vi "MultiChannelFeedbackCooling_aod_feedback(Host)_PIDXYZ_laserPID.vi"(5 "RIO Device":T1="RIO0") -> ()   [LabVIEW 2018]
doc: "This VI will will initialize the FPGA VI and then continually read and convert single point values from 4 channels of an analog input module."
uses:
  <vilib>/userdefined/High Color/nirio_resource_hc.ctl
  <vilib>/rvi/Analysis/host/Butterworth/config/Butterworth Filter Order.ctl
  <vilib>/rvi/Analysis/host/Butterworth/config/Butterworth Filter Type.ctl
  <vilib>/FPGAPlugInAG/PXIe-7856R/niLvFpga_Open_PXIe-7856R.vi
  <vilib>/FPGAPlugInAG/PXIe-7856R/niLvFpga_Run_PXIe-7856R.vi
  <vilib>/rvi/Analysis/host/Butterworth/config/BwScaledCoefficients.vi
  <vilib>/Utility/error.llb/Error Cluster From Error Code.vi
  <vilib>/rvi/errors/niLvFpgaAdjustHostInterfaceError.vi
  <vilib>/Utility/file.llb/Read From Spreadsheet File (I64).vi
  <vilib>/FPGAPlugInAG/PXIe-7856R/niLvFpga_Close_PXIe-7856R.vi
  <vilib>/rvi/interface/nirviOpenFPGA/nirviOpenFPGA.xnode
  FPGA Bitfiles/Microspherefeedb_FPGATarget2_MultiChannelfFee_SMENcAWM-fA.lvbitx
  <vilib>/rvi/interface/nirviMethod/nirviMethod.xnode
  <vilib>/rvi/Analysis/host/Butterworth/XNode/ButterworthCoefficients.xnode
  <vilib>/rvi/interface/nirviReadWriteControl/nirviReadWriteControl.xnode
  <vilib>/rvi/interface/nirviCloseFPGA/nirviCloseFPGA.xnode
  NiFpgaLv.dll
  <vilib>/rvi/Analysis/host/Public/NI_FpgaMspHost.lvlib
panel:
  in  "LP FF Z before":dbl=1000.0
  in  "LP FF Y before":dbl=1000.0
  in  "LP FF X Before":dbl=1000.0
  in  "LP FF Z":dbl=5000.0
  in  "LP FF Y":dbl=5000.0
  in  "LP FF X":dbl=5000.0
  in  "Lower lim Y before":fxp<+/-,16,16>=10000.0
  in  "Upper lim Y before":fxp<+/-,16,16>=10000.0
  in  "Lower lim X before":fxp<+/-,16,16>=10000.0
  in  "Upper lim X before":fxp<+/-,16,16>=10000.0
  in  "?":u16(ring)=2 items=["Both", "AOD", "Bead"]
  in  "?":u16(ring)=2 items=["Both", "AOD", "Bead"]
  out "Tot feedback + DC, Z":i16(graph)=16788
  out "Individual feedback, Z":cluster{"fb_0":i16, "fb_d0":i16}(graph)
  out "AI 2":cluster{"AI1":i16, "AI4":i16}(graph)={"AI1"=5242, "AI4"=5242}
  in  "Use PID Y before":bool
  in  "Use PID X before":bool
  in  "Ig Y before":fxp<+/-,24,12>
  in  "Dg Y before":fxp<+/-,24,12>
  in  "Pg Y before":fxp<+/-,24,12>
  in  "Ig X before":fxp<+/-,24,12>
  in  "Dg X before":fxp<+/-,24,12>
  in  "Pg X before":fxp<+/-,24,12>
  in  "Y before setpoint":i16
  in  "X before setpoint":i16
  in  "dg band X before":fxp<+/-,24,12>
  in  "dg band Y before":fxp<+/-,24,12>
  in  "hp freq X band before":dbl=5000.0
  in  "lp freq X band before":dbl=5000.0
  in  "hp freq X before":dbl=5000.0
  in  "lp freq X before":dbl=5000.0
  in  "hp freq Y band before":dbl=5000.0
  in  "lp freq Y band before":dbl=5000.0
  in  "hp freq Y before":dbl=5000.0
  in  "lp freq Y before":dbl=5000.0
  out "EOM_amplitude_out":dbl=4.999694842844065
  in  "EOM_offset (-10 to 10 V)":dbl
  in  "EOM_amplitude (-10 to 10 V)":dbl=5.0
  in  "EOM_threshold (0 to 1), (2*thr - 1)*ampli":dbl=1.0
  in  "EOM reset":bool
  in  "hp freq band Z before":dbl=5000.0
  in  "lp freq band Z before":dbl=5000.0
  in  "dg band Z before":fxp<+/-,24,12>
  in  "hp freq bandZ":dbl=49.0
  in  "lp freq bandZ":dbl=45.0
  in  "dg band Z":fxp<+/-,24,12>
  in  "dg band Y":fxp<+/-,24,12>
  in  "hp freq bandY":dbl=5000.0
  in  "lp freq bandY":dbl=5000.0
  in  "hp freq bandX":dbl=5000.0
  in  "lp freq bandX":dbl=5000.0
  in  "dg band X":fxp<+/-,24,12>
  in  "Pg Y":fxp<+/-,24,12>
  in  "Ig Y":fxp<+/-,24,6>
  in  "Pg X":fxp<+/-,24,12>
  in  "Ig X":fxp<+/-,24,6>
  in  "End value arb (ch1)":fxp<+/-,32,16>=1.0
  in  "Step arb (ch1)":fxp<+/-,32,16>=0.100006103515625
  in  "Arb gain (Z)":fxp<+/-,24,12>=1.0
  in  "z arb scale":fxp<+/-,33,17>=1.0
  in  "ramp arb drive":bool
  in  "End value arb (ch0)":fxp<+/-,32,16>=1.0
  in  "Step arb (ch0)":fxp<+/-,32,16>=1.0
  in  "Delay Time (s) arb":dbl=0.001 caption="Delay Time (s)"
  in  "Buffer file path":path=path "C:/Users/yalem/GitHub/Documents/Optlev/scriptssiny_buffer.txt"
  in  "Write data to buffers":bool
  in  "Arb steps per cycle":u16=20
  in  "Arb gain (Y)":fxp<+/-,24,12>
  in  "Arb gain (X)":fxp<+/-,24,12>
  in  "Z before setpoint":i16
  in  "Upper lim Z before":fxp<+/-,16,16>=10000.0
  in  "Lower lim Z before":fxp<+/-,16,16>=-10000.0
  in  "hp freq Z before":dbl=5000.0
  in  "lp freq Z before":dbl=5000.0
  in  "Use PID Z before":bool
  in  "hp freq Y":dbl=1300.0
  in  "hp freq X":dbl=1300.0
  in  "lp freq X":dbl=1300.0
  in  "DC offset X":i16=16310
  in  "Lower lim X":fxp<+/-,16,16>=-15000.0
  in  "Upper lim X":fxp<+/-,16,16>=15000.0
  in  "Dg X":fxp<+/-,24,12>
  in  "X setpoint":i16
  in  "change pars":bool
  in  "hp freq Z":dbl=1800.0
  in  "lp freq Y":dbl=1300.0
  in  "lp freq Z":dbl=1800.0
  in  "ramp power":bool
  in  "End value power":i16=10200
  in  "Step power":i16=4
  in  "Delay Time (s) power":dbl=0.01 caption="Delay Time (s)"
  in  "Count(usec)":u32=10
  in  "?":u16(ring)=2 items=["Both", "AOD", "Bead"]
  in  "?":u16(ring)=2 items=["Both", "AOD", "Bead"]
  in  "?":u16(ring)=2 items=["Both", "AOD", "Bead"]
  in  "?":u16(ring)=2 items=["Both", "AOD", "Bead"]
  in  "Pg Z before":fxp<+/-,24,12>
  in  "Ig Z before":fxp<+/-,24,6>
  in  "Dg Z before":fxp<+/-,24,12>
  in  "Ig Z":fxp<+/-,24,6>
  in  "DC offset Z":i16=16788
  in  "Lower lim Z":fxp<+/-,16,16>=-20.0
  in  "Upper lim Z":fxp<+/-,16,16>=1000.0
  in  "Dg Z":fxp<+/-,24,12>
  in  "Pg Z":fxp<+/-,24,12>
  in  "Z setpoint":i16
  in  "change pars 2":bool
  in  "change pars 1":bool
  in  "DC offset Y":i16=16310
  in  "Lower lim Y":fxp<+/-,16,16>=-15000.0
  in  "Upper lim Y":fxp<+/-,16,16>=15000.0
  in  "Dg Y":fxp<+/-,24,12>
  in  "Y setpoint":i16
  out "Tot feedback + DC, Y":i16(graph)=16310
  out "Individual feedback, Y":cluster{"fb_0":i16, "fb_d0":i16}(graph)
  out "AI1":cluster{"AI1":i16, "AI4":i16}(graph)={"AI1"=-2712, "AI4"=-2712}
  out "Tot feedback + DC, X":i16(graph)=16309
  out "Individual feedback, X":cluster{"fb_0":i16, "fb_d0":i16}(graph)
  out "AI0":cluster{"AI0":i16, "AI3":i16}(graph)={"AI0"=-863, "AI3"=-863}
  in  "stop":bool
  # "FPGA feedback GUI"
  # "Bead arbitrary drive:"
  # "PID controls, X (ch 0):"
  # "Bead feedback:"
  # "PID controls, Y (ch 1):"
  # "Bead feedback:"
  # "PID controls, Z (ch 2):"
  # "Bead feedback:"
  # "AOD feeback:"
types:
  T1 = typedef "nirio_resource_hc.ctl" = tag
  T2 = cluster{"fb Z plot":i16, "fb Z before chamber plot":i16}
  T3 = cluster{"fb Z before chamber plot":i16, "fb Z before chamber plot":i16}
  T4 = cluster{"AI Z plot":i16, "AI Z before chamber plot":i16}
  T5 = cluster{"AI Z before chamber plot":i16, "AI Z before chamber plot":i16}
  T6 = cluster{"AI X plot":i16, "AI X before chamber plot":i16}
  T7 = cluster{"AI X before chamber plot":i16, "AI X before chamber plot":i16}
  T8 = cluster{"fb X plot":i16, "fb X before chamber plot":i16}
  T9 = cluster{"fb X before chamber plot":i16, "fb X before chamber plot":i16}
  T10 = cluster{"fb Y plot":i16, "fb Y before chamber plot":i16}
  T11 = cluster{"fb Y before chamber plot":i16, "fb Y before chamber plot":i16}
  T12 = cluster{"AI Y plot":i16, "AI Y before chamber plot":i16}
  T13 = cluster{"AI Y before chamber plot":i16, "AI Y before chamber plot":i16}
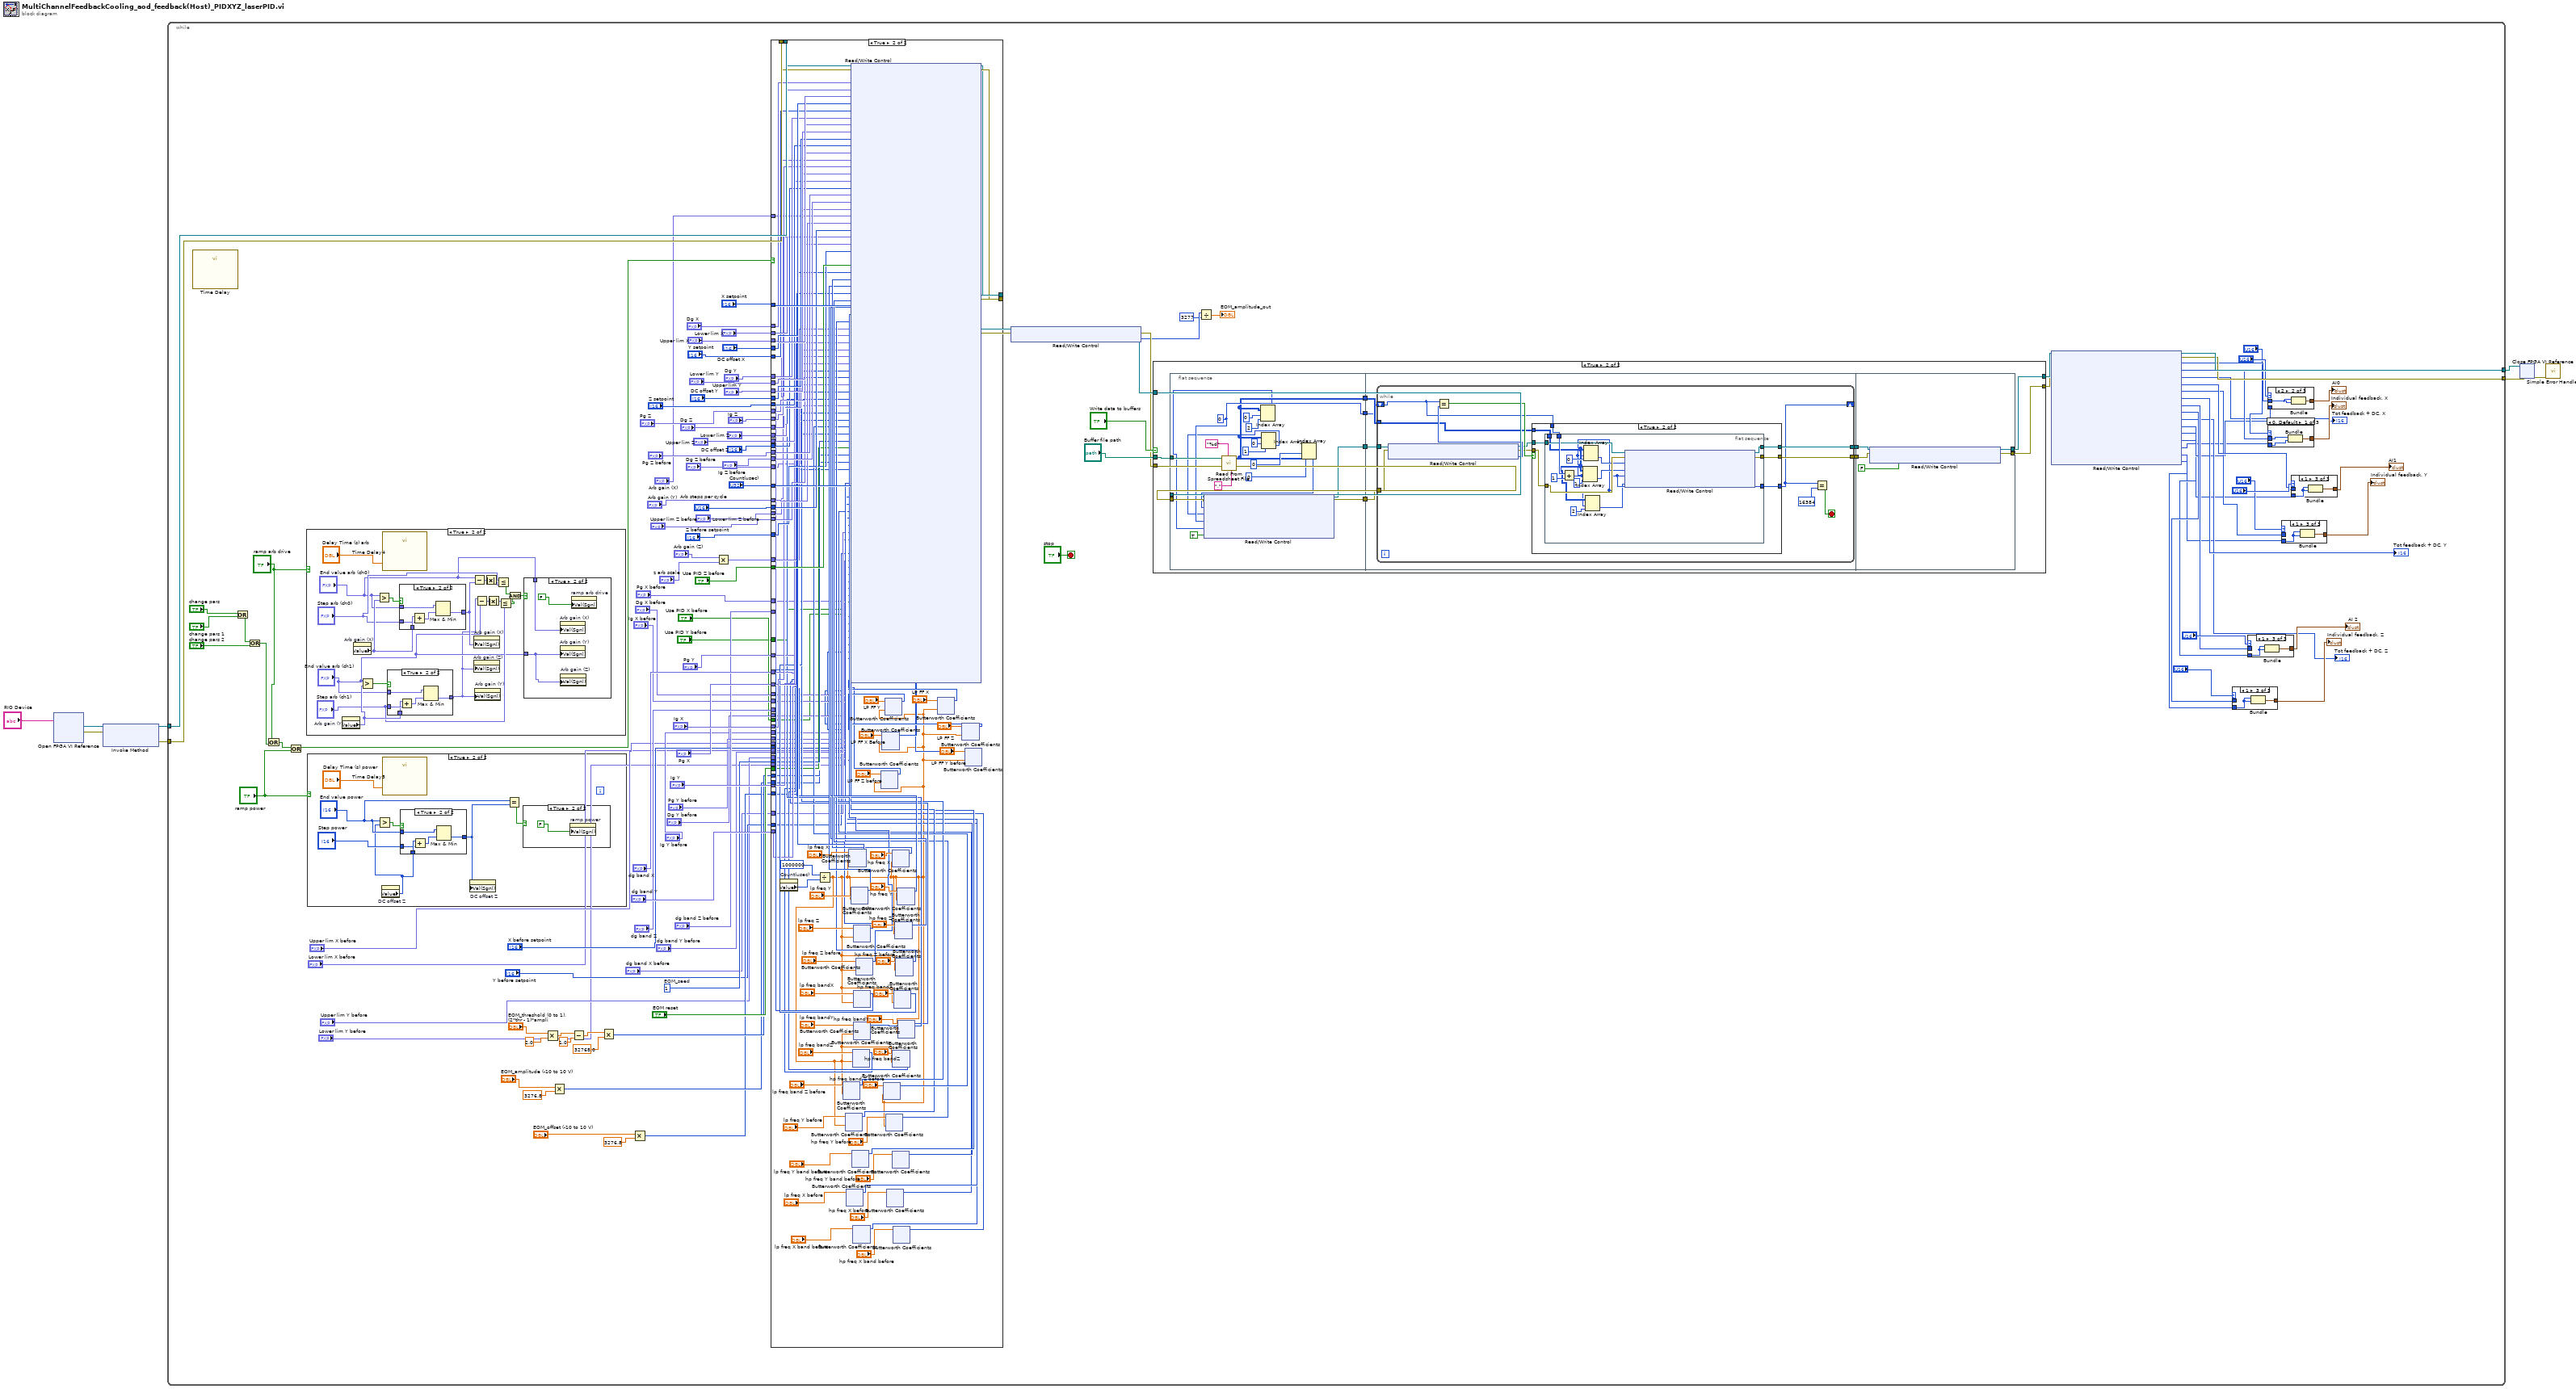
[diagram p0: block diagram]
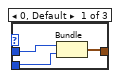
[diagram p2: hidden frame]
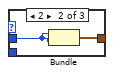
[diagram p3: hidden frame]
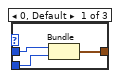
[diagram p4: hidden frame]
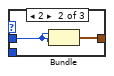
[diagram p5: hidden frame]
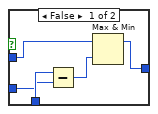
[diagram p8: hidden frame]
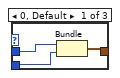
[diagram p9: hidden frame]
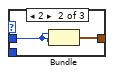
[diagram p10: hidden frame]
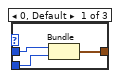
[diagram p11: hidden frame]
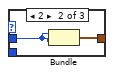
[diagram p12: hidden frame]
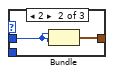
[diagram p13: hidden frame]
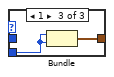
[diagram p14: hidden frame]
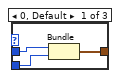
[diagram p15: hidden frame]
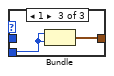
[diagram p16: hidden frame]
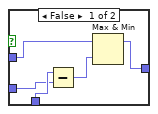
[diagram p18: hidden frame]
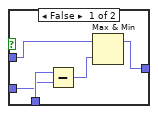
[diagram p20: hidden frame]
diagram:
  n1 = xnode "Open FPGA VI Reference"("resource name"="RIO Device") -> ("FPGA VI Reference Out"=w3:refnum<k20>, "error out"=w2:errorcluster)  [unwired: 1 in]
  n2 = xnode "Invoke Method"("FPGA VI Reference In"=w3, "error in"=w2) -> ("FPGA VI Reference Out"=w5:refnum<k20>, "error out"=w4:errorcluster)  [unwired: 1 in]
  n3 = while {
    tunnel: [w130] -> w8
    tunnel: w5 -> [w122]
    tunnel: w4 -> [w121]
    tunnel: [w129] -> w1
    stop <- "stop" stop-if-true
    w60 = u32 1  # EOM_seed
    n4 = call "Time Delay"() -> ()  [unwired: 11 in, 1 out]
    n5 = Or(x="change pars", y="change pars 1") -> (x .or. y?=w97:bool)
    n6 = Or(x=w97, y="change pars 2") -> (x .or. y?=w73:bool)
    n7 = Or(x="ramp arb drive", y=w73) -> (x .or. y?=w80:bool)
    n8 = Or(x=w80, y="ramp power") -> (x .or. y?=w81:bool)
    n9 = case shown="True" "ramp arb drive" {
      frame False {
      }
      frame True {
        n10 = property on="Arb gain (Y)" class="DigNum (strict)"() -> ("Value"=w204:fxp<+/-,24,12>)  [unwired: 2 in, 2 out]
        n11 = property on="Arb gain (X)" class="DigNum (strict)"() -> ("Value"=w207:fxp<+/-,24,12>)  [unwired: 2 in, 2 out]
        n12 = Greater?(x="End value arb (ch1)", y=w204) -> (0:w205:bool)
        n13 = Greater?(x="End value arb (ch0)", y=w207) -> (0:w208:bool)
        n14 = call "Time Delay4"("Delay Time (s)"="Delay Time (s) arb") -> ()  [unwired: 10 in, 1 out]
        n15 = case shown="True" w205 {
          tunnel: "End value arb (ch1)" -> [w210 w216]
          tunnel: w204 -> [w213 w214]
          tunnel: "Step arb (ch1)" -> [w212 w218]
          tunnel: [w209 w215] -> w191
          frame False {
            n16 = Subtract(x=w213, y=w212) -> (x-y=w211:fxp<+/-,33,17>)
            n17 = Max & Min(x=w210, y=w211) -> (max(x,y)=w209:fxp<+/-,33,17>)  [unwired: 1 out]
          }
          frame True {
            n18 = Add(x=w214, y=w218) -> (x+y=w217:fxp<+/-,33,17>)
            n19 = Max & Min(x=w216, y=w217) -> (min(x,y)=w215:fxp<+/-,33,17>)  [unwired: 1 out]
          }
        }
        n20 = case shown="True" w208 {
          tunnel: "End value arb (ch0)" -> [w223 w228]
          tunnel: w207 -> [w226 w231]
          tunnel: "Step arb (ch0)" -> [w225 w230]
          tunnel: [w222 w227] -> w203
          frame False {
            n21 = Subtract(x=w226, y=w225) -> (x-y=w224:fxp<+/-,33,17>)
            n22 = Max & Min(x=w223, y=w224) -> (max(x,y)=w222:fxp<+/-,33,17>)  [unwired: 1 out]
          }
          frame True {
            n23 = Add(x=w231, y=w230) -> (x+y=w229:fxp<+/-,33,17>)
            n24 = Max & Min(x=w228, y=w229) -> (min(x,y)=w227:fxp<+/-,33,17>)  [unwired: 1 out]
          }
        }
        n25 = Subtract(x="End value arb (ch0)", y=w203) -> (x-y=w202:fxp<+/-,34,18>)
        n26 = property on="Arb gain (X)" class="DigNum (strict)"("Val(Sgnl)"=w203) -> ()  [unwired: 2 in, 2 out]
        n27 = property on="Arb gain (Z)" class="DigNum (strict)"("Val(Sgnl)"=w191) -> ()  [unwired: 2 in, 2 out]
        n28 = Subtract(x=w191, y="End value arb (ch1)") -> (x-y=w199:fxp<+/-,34,18>)
        n29 = property on="Arb gain (Y)" class="DigNum (strict)"("Val(Sgnl)"=w191) -> ()  [unwired: 2 in, 2 out]
        n30 = Absolute Value(x=w202) -> (abs(x)=w201:fxp<+,33,17>)
        n31 = Absolute Value(x=w199) -> (abs(x)=w198:fxp<+,33,17>)
        n32 = Less Or Equal?(x=w201, y="Step arb (ch0)") -> (x <= y?=w195:bool)
        n33 = Less Or Equal?(x=w198, y="Step arb (ch1)") -> (x <= y?=w194:bool)
        n34 = And(x=w195, y=w194) -> (x .and. y?=w196:bool)
        n35 = case shown="True" w196 {
          tunnel: "End value arb (ch0)" -> [_ w220]
          tunnel: "End value arb (ch1)" -> [_ w219]
          frame False {
          }
          frame True {
            n36 = property on="Arb gain (X)" class="DigNum (strict)"("Val(Sgnl)"=w220) -> ()  [unwired: 2 in, 2 out]
            n37 = property on="Arb gain (Y)" class="DigNum (strict)"("Val(Sgnl)"=w219) -> ()  [unwired: 2 in, 2 out]
            n38 = property on="Arb gain (Z)" class="DigNum (strict)"("Val(Sgnl)"=w219) -> ()  [unwired: 2 in, 2 out]
            n39 = property on="ramp arb drive" class="Bool (strict)"("Val(Sgnl)"=FALSE) -> ()  [unwired: 2 in, 2 out]
          }
        }
      }
    }
    n40 = case shown="True" "ramp power" {
      frame False {
      }
      frame True {
        n41 = property on="DC offset Z" class="DigNum (strict)"() -> ("Value"=w146:i16)  [unwired: 2 in, 2 out]
        n42 = Greater?(x="End value power", y=w146) -> (0:w151:bool)
        n43 = call "Time Delay5"("Delay Time (s)"="Delay Time (s) power") -> ()  [unwired: 10 in, 1 out]
        n44 = case shown="True" w151 {
          tunnel: "End value power" -> [w154 w159]
          tunnel: w146 -> [w157 w162]
          tunnel: "Step power" -> [w156 w161]
          tunnel: [w153 w158] -> w145
          frame False {
            n45 = Subtract(x=w157, y=w156) -> (x-y=w155:i16)
            n46 = Max & Min(x=w154, y=w155) -> (max(x,y)=w153:i16)  [unwired: 1 out]
          }
          frame True {
            n47 = Add(x=w162, y=w161) -> (x+y=w160:i16)
            n48 = Max & Min(x=w159, y=w160) -> (min(x,y)=w158:i16)  [unwired: 1 out]
          }
        }
        n49 = property on="DC offset Z" class="DigNum (strict)"("Val(Sgnl)"=w145) -> ()  [unwired: 2 in, 2 out]
        n50 = Equal?(x="End value power", y=w145) -> (x = y?=w150:bool)
        n51 = case shown="True" w150 {
          frame False {
          }
          frame True {
            n52 = property on="ramp power" class="Bool (strict)"("Val(Sgnl)"=FALSE) -> ()  [unwired: 2 in, 2 out]
          }
        }
      }
    }
    n53 = Multiply(x="EOM_threshold (0 to 1), (2*thr - 1)*ampli", y=2.0) -> (x*y=w56:dbl)
    n54 = Multiply(x="EOM_amplitude (-10 to 10 V)", y=3276.8) -> (x*y=w49:i16)
    n55 = Subtract(x=w56, y=1.0) -> (x-y=w54:dbl)
    n56 = Multiply(x=w54, y=32768.0) -> (x*y=w52:i16)
    n57 = Multiply(x="EOM_offset (-10 to 10 V)", y=3276.8) -> (x*y=w46:i16)
    n58 = Multiply(x="Arb gain (Z)", y="z arb scale") -> (x*y=w70:fxp<+/-,56,28>)
    n59 = case shown="True" w81 {
      tunnel: w121 -> [w313 w429]
      tunnel: [w313 w437] -> w45
      tunnel: [w312 w436] -> w44
      tunnel: "X setpoint" -> [_ w435]
      tunnel: "Dg X" -> [_ w434]
      tunnel: "Upper lim X" -> [_ w432]
      tunnel: "Lower lim X" -> [_ w433]
      tunnel: "DC offset X" -> [_ w431]
      tunnel: w122 -> [w312 w430]
      tunnel: "Y setpoint" -> [_ w428]
      tunnel: "Dg Y" -> [_ w427]
      tunnel: "Lower lim Y" -> [_ w426]
      tunnel: "Upper lim Y" -> [_ w425]
      tunnel: "DC offset Y" -> [_ w424]
      tunnel: "Z setpoint" -> [_ w423]
      tunnel: "Pg Z" -> [_ w422]
      tunnel: "Ig Z" -> [_ w421]
      tunnel: "Dg Z" -> [_ w420]
      tunnel: "Lower lim Z" -> [_ w419]
      tunnel: "Upper lim Z" -> [_ w418]
      tunnel: "DC offset Z" -> [_ w417]
      tunnel: "Pg Z before" -> [_ w416]
      tunnel: "Ig Z before" -> [_ w415]
      tunnel: "Dg Z before" -> [_ w360]
      tunnel: "Arb gain (Y)" -> [_ w401]
      tunnel: "Arb steps per cycle" -> [_ w414]
      tunnel: "Count(usec)" -> [_ w413]
      tunnel: "Use PID Z before" -> [_ w404]
      tunnel: "Lower lim Z before" -> [_ w400]
      tunnel: "Upper lim Z before" -> [_ w399]
      tunnel: "Z before setpoint" -> [_ w398]
      tunnel: w70 -> [_ w389]
      tunnel: "Ig X" -> [_ w388]
      tunnel: "Pg X" -> [_ w387]
      tunnel: "Ig Y" -> [_ w386]
      tunnel: "Pg Y" -> [_ w385]
      tunnel: "dg band X" -> [_ w384]
      tunnel: "dg band Y" -> [_ w377]
      tunnel: "dg band Z" -> [_ w374]
      tunnel: "dg band Z before" -> [_ _]
      tunnel: w60 -> [_ w365]
      tunnel: "EOM reset" -> [_ w364]
      tunnel: w52 -> [_ w363]
      tunnel: w49 -> [_ w362]
      tunnel: w46 -> [_ w361]
      tunnel: "dg band Y before" -> [_ w343]
      tunnel: "dg band X before" -> [_ w342]
      tunnel: "X before setpoint" -> [_ w341]
      tunnel: "Y before setpoint" -> [_ w340]
      tunnel: "Pg X before" -> [_ w339]
      tunnel: "Dg X before" -> [_ w338]
      tunnel: "Ig X before" -> [_ w337]
      tunnel: "Pg Y before" -> [_ w336]
      tunnel: "Dg Y before" -> [_ w335]
      tunnel: "Ig Y before" -> [_ w334]
      tunnel: "Use PID X before" -> [_ w333]
      tunnel: "Use PID Y before" -> [_ w332]
      tunnel: "Upper lim X before" -> [_ w331]
      tunnel: "Lower lim X before" -> [_ w330]
      tunnel: "Upper lim Y before" -> [_ w329]
      tunnel: "Lower lim Y before" -> [_ w328]
      tunnel: "Arb gain (X)" -> [_ w314]
      frame False {
      }
      frame True {
        n60 = property on="Count(usec)" class="DigNum (strict)"() -> ("Value"=w409:u32)  [unwired: 2 in, 2 out]
        n61 = Divide(x=u32 1000000, y=w409) -> (x/y=w316:dbl)
        n62 = xnode "Butterworth Coefficients"("cutoff frequency (Hz)"="lp freq band Z before", "sample rate (S/s)"=w316) -> ("scaled coefficients"=w366:i32[])  [unwired: 1 in, 1 out]
        n63 = xnode "Butterworth Coefficients"("cutoff frequency (Hz)"="lp freq Y before", "sample rate (S/s)"=w316) -> ("scaled coefficients"=w357:i32[])  [unwired: 1 in, 1 out]
        n64 = xnode "Butterworth Coefficients"("cutoff frequency (Hz)"="lp freq X before") -> ("scaled coefficients"=w347:i32[])  [unwired: 2 in, 1 out]
        n65 = xnode "Butterworth Coefficients"("cutoff frequency (Hz)"="lp freq X", "sample rate (S/s)"=w316) -> ("scaled coefficients"=w397:i32[])  [unwired: 1 in, 1 out]
        n66 = xnode "Butterworth Coefficients"("cutoff frequency (Hz)"="lp freq Y", "sample rate (S/s)"=w316) -> ("scaled coefficients"=w395:i32[])  [unwired: 1 in, 1 out]
        n67 = xnode "Butterworth Coefficients"("cutoff frequency (Hz)"="lp freq Y band before") -> ("scaled coefficients"=w353:i32[])  [unwired: 2 in, 1 out]
        n68 = xnode "Butterworth Coefficients"("cutoff frequency (Hz)"="lp freq bandZ", "sample rate (S/s)"=w316) -> ("scaled coefficients"=w370:i32[])  [unwired: 1 in, 1 out]
        n69 = xnode "Butterworth Coefficients"("cutoff frequency (Hz)"="lp freq X band before") -> ("scaled coefficients"=w345:i32[])  [unwired: 2 in, 1 out]
        n70 = xnode "Butterworth Coefficients"("cutoff frequency (Hz)"="lp freq Z", "sample rate (S/s)"=w316) -> ("scaled coefficients"=w393:i32[])  [unwired: 1 in, 1 out]
        n71 = xnode "Butterworth Coefficients"("cutoff frequency (Hz)"="lp freq bandX", "sample rate (S/s)"=w316) -> ("scaled coefficients"=w380:i32[])  [unwired: 1 in, 1 out]
        n72 = xnode "Butterworth Coefficients"("cutoff frequency (Hz)"="lp freq bandY", "sample rate (S/s)"=w316) -> ("scaled coefficients"=w376:i32[])  [unwired: 1 in, 1 out]
        n73 = xnode "Butterworth Coefficients"("cutoff frequency (Hz)"="lp freq Z before", "sample rate (S/s)"=w316) -> ("scaled coefficients"=w391:i32[])  [unwired: 1 in, 1 out]
        n74 = xnode "Butterworth Coefficients"("cutoff frequency (Hz)"="LP FF Z before", "sample rate (S/s)"=w316) -> ("scaled coefficients"=w315:i32[])  [unwired: 1 in, 1 out]
        n75 = xnode "Butterworth Coefficients"("cutoff frequency (Hz)"="LP FF X Before", "sample rate (S/s)"=w316) -> ("scaled coefficients"=w320:i32[])  [unwired: 1 in, 1 out]
        n76 = xnode "Butterworth Coefficients"("cutoff frequency (Hz)"="hp freq band Z before", "sample rate (S/s)"=w316) -> ("scaled coefficients"=w367:i32[])  [unwired: 1 in, 1 out]
        n77 = xnode "Butterworth Coefficients"("cutoff frequency (Hz)"="LP FF Y", "sample rate (S/s)"=w316) -> ("scaled coefficients"=w324:i32[])  [unwired: 1 in, 1 out]
        n78 = xnode "Butterworth Coefficients"("cutoff frequency (Hz)"="hp freq Y before", "sample rate (S/s)"=w316) -> ("scaled coefficients"=w356:i32[])  [unwired: 1 in, 1 out]
        n79 = xnode "Butterworth Coefficients"("cutoff frequency (Hz)"="hp freq X before") -> ("scaled coefficients"=w346:i32[])  [unwired: 2 in, 1 out]
        n80 = xnode "Butterworth Coefficients"("cutoff frequency (Hz)"="hp freq X", "sample rate (S/s)"=w316) -> ("scaled coefficients"=w396:i32[])  [unwired: 1 in, 1 out]
        n81 = xnode "Butterworth Coefficients"("cutoff frequency (Hz)"="hp freq Y band before") -> ("scaled coefficients"=w352:i32[])  [unwired: 2 in, 1 out]
        n82 = xnode "Butterworth Coefficients"("cutoff frequency (Hz)"="hp freq bandZ", "sample rate (S/s)"=w316) -> ("scaled coefficients"=w371:i32[])  [unwired: 1 in, 1 out]
        n83 = xnode "Butterworth Coefficients"("cutoff frequency (Hz)"="hp freq X band before") -> ("scaled coefficients"=w344:i32[])  [unwired: 2 in, 1 out]
        n84 = xnode "Butterworth Coefficients"("cutoff frequency (Hz)"="hp freq bandX", "sample rate (S/s)"=w316) -> ("scaled coefficients"=w381:i32[])  [unwired: 1 in, 1 out]
        n85 = xnode "Butterworth Coefficients"("cutoff frequency (Hz)"="hp freq Z", "sample rate (S/s)"=w316) -> ("scaled coefficients"=w392:i32[])  [unwired: 1 in, 1 out]
        n86 = xnode "Butterworth Coefficients"("cutoff frequency (Hz)"="hp freq Z before", "sample rate (S/s)"=w316) -> ("scaled coefficients"=w390:i32[])  [unwired: 1 in, 1 out]
        n87 = xnode "Butterworth Coefficients"("cutoff frequency (Hz)"="hp freq Y", "sample rate (S/s)"=w316) -> ("scaled coefficients"=w394:i32[])  [unwired: 1 in, 1 out]
        n88 = xnode "Butterworth Coefficients"("cutoff frequency (Hz)"="hp freq bandY", "sample rate (S/s)"=w316) -> ("scaled coefficients"=w375:i32[])  [unwired: 1 in, 1 out]
        n89 = xnode "Butterworth Coefficients"("cutoff frequency (Hz)"="LP FF X", "sample rate (S/s)"=w316) -> ("scaled coefficients"=w326:i32[])  [unwired: 1 in, 1 out]
        n90 = xnode "Butterworth Coefficients"("cutoff frequency (Hz)"="LP FF Z", "sample rate (S/s)"=w316) -> ("scaled coefficients"=w322:i32[])  [unwired: 1 in, 1 out]
        n91 = xnode "Butterworth Coefficients"("cutoff frequency (Hz)"="LP FF Y before", "sample rate (S/s)"=w316) -> ("scaled coefficients"=w318:i32[])  [unwired: 1 in, 1 out]
        n92 = xnode "Read/Write Control"("FPGA VI Reference In"=w430, "error in"=w429, "X Setpoint"=w435, "dg X"=w434, "Lower lim X"=w433, "Upper lim X"=w432, "DC offset X"=w431, "Y Setpoint"=w428, "dg Y"=w427, "Lower lim Y"=w426, "Upper lim Y"=w425, "DC offset Y"=w424, "Z Setpoint"=w423, "pg Z"=w422, "ig Z"=w421, "dg Z"=w420, "Lower lim Z"=w419, "Upper lim Z"=w418, "DC offset Z"=w417, "pg Z before"=w416, "ig Z before"=w415, "dg Z before"=w360, "Arb gain (ch0)"=w314, "Arb gain (ch1)"=w401, "Arb steps per cycle"=w414, "Lower lim Z before"=w400, "Upper lim Z before"=w399, "Z before Setpoint"=w398, "Count(uSec)"=w413, "Use Z PID before"=w404, "LP Coeff X"=w397, "HP Coeff X"=w396, "LP Coeff Y"=w395, "HP Coeff Y"=w394, "LP Coeff Z"=w393, "HP Coeff Z"=w392, "LP Coeff band Z before"=w391, "HP coeff band Z before"=w390, "Arb gain (ch2)"=w389, "ig X"=w388, "pg X"=w387, "ig Y"=w386, "pg Y"=w385, "dg band X"=w384, "HP Coeff band X"=w381, "LP Coeff band X"=w380, "dg band Y"=w377, "HP Coeff band Y"=w375, "LP Coeff band Y"=w376, "dg band Z"=w374, "HP Coeff band Z"=w371, "LP Coeff band Z"=w370, "HP Coeff band Z"=w367, "LP Coeff band Z"=w366, "EOM_seed"=w365, "EOM reset"=w364, "EOM_threshold"=w363, "EOM_amplitude"=w362, "EOM_offset"=w361, "LP Coeff Y before"=w357, "HP Coeff Y before"=w356, "LP Coeff band Y before"=w353, "HP coeff band Y before"=w352, "LP Coeff X before"=w347, "HP Coeff X before"=w346, "LP Coeff band X before"=w345, "HP coeff band X before"=w344, "dg band Y before"=w343, "dg band X before"=w342, "X before Setpoint"=w341, "Y before Setpoint"=w340, "pg X before"=w339, "dg X before"=w338, "ig X before"=w337, "pg Y before"=w336, "dg Y before"=w335, "ig Y before"=w334, "Use X PID before"=w333, "Use Y PID before"=w332, "Upper lim X before"=w331, "Lower lim X before"=w330, "Upper lim Y before"=w329, "Lower lim Y before"=w328, "final filter coeff X"=w326, "final filter coeff Y"=w324, "final filter coeff Z"=w322, "final filter coeff X before"=w320, "final filter coeff Y before"=w318, "final filter coeff Z before"=w315) -> ("FPGA VI Reference Out"=w436:refnum<k20>, "error out"=w437:errorcluster)
      }
    }
    n93 = xnode "Read/Write Control"("FPGA VI Reference In"=w44, "error in"=w45) -> ("FPGA VI Reference Out"=w43:refnum<k20>, "error out"=w42:errorcluster, "EOM_amplitude"=w41:i16)
    n94 = case shown="True" "Write data to buffers" {
      tunnel: "Buffer file path" -> [_ w244]
      tunnel: w43 -> [w233 w243]
      tunnel: w42 -> [w232 w242]
      tunnel: [w233 w235] -> w118
      tunnel: [w232 w234] -> w117
      frame False {
      }
      frame True {
        n95 = flat-sequence {
          tunnel: w244 -> [w263]
          tunnel: w243 -> [w261]
          tunnel: w242 -> [w260]
          tunnel: [w255] -> w241
          tunnel: [w254] -> w240
          tunnel: [w248] -> w239
          tunnel: [w253] -> w238
          tunnel: w241 -> [w269]
          tunnel: w240 -> [w268]
          tunnel: w239 -> [w267]
          tunnel: w238 -> [w266]
          tunnel: [w265] -> w237
          tunnel: [w264] -> w236
          tunnel: w237 -> [w311]
          tunnel: w236 -> [w310]
          tunnel: [w309] -> w235
          tunnel: [w308] -> w234
          frame #0 {
            w253 = 0
            n96 = call-poly <vilib>:"Read From Spreadsheet File.vi"("delimiter (\\t)"="," ("delimiter (\\t)"), "format (%d)"="%d", "file path (dialog if empty)"=w263) -> ("all rows"=w248:i64[][])  [unwired: 4 in, 4 out]
            n97 = Index Array(array=w248, index (row)=0, index (col)=2 ("disabled index (col)")) -> (element=w245:i64)
            n98 = Index Array(array=w248, index (row)=0, index (col)=1 ("disabled index (col)")) -> (element=w251:i64)
            n99 = Index Array(array=w248, index (row)=0, index (col)=0 ("disabled index (col)")) -> (element=w252:i64)
            n100 = xnode "Read/Write Control"("FPGA VI Reference In"=w261, "error in"=w260, "data_buffer_1"=w252, "data_buffer2"=w251, "write_address"=w253, "data_buffer3"=w245, "ready_to_write"=TRUE) -> ("FPGA VI Reference Out"=w254:refnum<k20>, "error out"=w255:errorcluster)
          }
          frame #1 {
            n101 = while {
              shift-right: [w270] -> _
              shift-left: w266 -> [w278]
              tunnel: w268 -> [w282]
              tunnel: w269 -> [w281]
              tunnel: w267 -> [w277]
              tunnel: [w272] -> w265
              tunnel: [w271] -> w264
              stop <- w273 stop-if-true
              n102 = xnode "Read/Write Control"("FPGA VI Reference In"=w282, "error in"=w281) -> ("FPGA VI Reference Out"=w276:refnum<k20>, "error out"=w275:errorcluster, "written_address"=w280:u32)
              n103 = Equal?(x=w278, y=w280) -> (x = y?=w279:bool)
              n104 = case shown="True" w279 {
                tunnel: w278 -> [w285 w292]
                tunnel: w277 -> [_ w291]
                tunnel: w276 -> [w284 w290]
                tunnel: w275 -> [w283 w289]
                tunnel: [w285 w288] -> w270
                tunnel: [w284 w287] -> w272
                tunnel: [w283 w286] -> w271
                frame False {
                }
                frame True {
                  n105 = flat-sequence {
                    tunnel: w292 -> [w305]
                    tunnel: w291 -> [w295]
                    tunnel: w290 -> [w302]
                    tunnel: w289 -> [w301]
                    tunnel: [w294] -> w288
                    tunnel: [w299] -> w287
                    tunnel: [w298] -> w286
                    frame #0 {
                      n106 = Add(x=w305, y=1) -> (x+y=w294:i32)
                      n107 = Index Array(array=w295, index (row)=w294, index (col)=1 ("disabled index (col)")) -> (element=w300:i64)
                      n108 = Index Array(array=w295, index (row)=w294, index (col)=0 ("disabled index (col)")) -> (element=w297:i64)
                      n109 = Index Array(array=w295, index (row)=w294, index (col)=2) -> (element=w293:i64)
                      n110 = xnode "Read/Write Control"("FPGA VI Reference In"=w302, "error in"=w301, "data_buffer_1"=w297, "data_buffer2"=w300, "write_address"=w294, "data_buffer3"=w293) -> ("FPGA VI Reference Out"=w299:refnum<k20>, "error out"=w298:errorcluster)
                    }
                  }
                }
              }
              n111 = Equal?(x=w270, y=u16 16384) -> (x = y?=w273:bool)
            }
          }
          frame #2 {
            n112 = xnode "Read/Write Control"("FPGA VI Reference In"=w311, "error in"=w310, "ready_to_write"=FALSE) -> ("FPGA VI Reference Out"=w309:refnum<k20>, "error out"=w308:errorcluster)
          }
        }
      }
    }
    n113 = Divide(x=w41, y=i16 3277) -> (x/y=→"EOM_amplitude_out":dbl)
    n114 = xnode "Read/Write Control"("FPGA VI Reference In"=w118, "error in"=w117) -> ("FPGA VI Reference Out"=w130:refnum<k20>, "error out"=w129:errorcluster, "AI X plot"=w95:i16, "fb X plot"=w90:i16, "tot_fb X plot"=→"Tot feedback + DC, X":i16, "AI Y plot"=w87:i16, "fb Y plot"=w85:i16, "tot_fb Y plot"=→"Tot feedback + DC, Y":i16, "AI Z plot"=w22:i16, "fb Z plot"=w21:i16, "tot_fb Z plot"=→"Tot feedback + DC, Z":i16, "AI X before chamber plot"=w19:i16, "AI Y before chamber plot"=w18:i16, "AI Z before chamber plot"=w17:i16, "fb X before chamber plot"=w16:i16, "fb Y before chamber plot"=w15:i16, "fb Z before chamber plot"=w14:i16)
    n115 = case shown="1" "?" {
      tunnel: w21 -> [w132 w134 _]
      tunnel: [w133 w135 w137] -> w24
      tunnel: w14 -> [w131 _ w136]
      frame 0, Default {
        n116 = Bundle("fb Z plot"=w132, "fb Z before chamber plot"=w131) -> (w133:T2)  [unwired: 1 in]
      }
      frame 2 {
        n117 = Bundle("fb Z plot"=w134, "fb Z plot"=w134) -> (w135:cluster{"fb Z plot":i16, "fb Z plot":i16})  [unwired: 1 in]
      }
      frame 1 {
        n118 = Bundle("fb Z before chamber plot"=w136, "fb Z before chamber plot"=w136) -> (w137:T3)  [unwired: 1 in]
      }
    }
    "Individual feedback, Z" <- w24
    n119 = case shown="1" "?" {
      tunnel: w22 -> [w139 w141 _]
      tunnel: [w140 w142 w144] -> w23
      tunnel: w17 -> [w138 _ w143]
      frame 0, Default {
        n120 = Bundle("AI Z plot"=w139, "AI Z before chamber plot"=w138) -> (w140:T4)  [unwired: 1 in]
      }
      frame 2 {
        n121 = Bundle("AI Z plot"=w141, "AI Z plot"=w141) -> (w142:cluster{"AI Z plot":i16, "AI Z plot":i16})  [unwired: 1 in]
      }
      frame 1 {
        n122 = Bundle("AI Z before chamber plot"=w143, "AI Z before chamber plot"=w143) -> (w144:T5)  [unwired: 1 in]
      }
    }
    "AI 2" <- w23
    n123 = case shown="2" "?" {
      tunnel: w95 -> [w186 w187 _]
      tunnel: [w185 w188 w190] -> w94
      tunnel: w19 -> [w184 _ w189]
      frame 0, Default {
        n124 = Bundle("AI X plot"=w186, "AI X before chamber plot"=w184) -> (w185:T6)  [unwired: 1 in]
      }
      frame 2 {
        n125 = Bundle("AI X plot"=w187, "AI X plot"=w187) -> (w188:cluster{"AI X plot":i16, "AI X plot":i16})  [unwired: 1 in]
      }
      frame 1 {
        n126 = Bundle("AI X before chamber plot"=w189, "AI X before chamber plot"=w189) -> (w190:T7)  [unwired: 1 in]
      }
    }
    "AI0" <- w94
    n127 = case shown="0, Default" "?" {
      tunnel: w90 -> [w179 w180 _]
      tunnel: [w178 w181 w183] -> w92
      tunnel: w16 -> [w177 _ w182]
      frame 0, Default {
        n128 = Bundle("fb X plot"=w179, "fb X before chamber plot"=w177) -> (w178:T8)  [unwired: 1 in]
      }
      frame 2 {
        n129 = Bundle("fb X plot"=w180, "fb X plot"=w180) -> (w181:cluster{"fb X plot":i16, "fb X plot":i16})  [unwired: 1 in]
      }
      frame 1 {
        n130 = Bundle("fb X before chamber plot"=w182, "fb X before chamber plot"=w182) -> (w183:T9)  [unwired: 1 in]
      }
    }
    "Individual feedback, X" <- w92
    n131 = case shown="1" "?" {
      tunnel: w85 -> [w164 w166 _]
      tunnel: [w165 w167 w169] -> w84
      tunnel: w15 -> [w163 _ w168]
      frame 0, Default {
        n132 = Bundle("fb Y plot"=w164, "fb Y before chamber plot"=w163) -> (w165:T10)  [unwired: 1 in]
      }
      frame 2 {
        n133 = Bundle("fb Y plot"=w166, "fb Y plot"=w166) -> (w167:cluster{"fb Y plot":i16, "fb Y plot":i16})  [unwired: 1 in]
      }
      frame 1 {
        n134 = Bundle("fb Y before chamber plot"=w168, "fb Y before chamber plot"=w168) -> (w169:T11)  [unwired: 1 in]
      }
    }
    "Individual feedback, Y" <- w84
    n135 = case shown="1" "?" {
      tunnel: w87 -> [w171 w173 _]
      tunnel: [w172 w174 w176] -> w82
      tunnel: w18 -> [w170 _ w175]
      frame 0, Default {
        n136 = Bundle("AI Y plot"=w171, "AI Y before chamber plot"=w170) -> (w172:T12)  [unwired: 1 in]
      }
      frame 2 {
        n137 = Bundle("AI Y plot"=w173, "AI Y plot"=w173) -> (w174:cluster{"AI Y plot":i16, "AI Y plot":i16})  [unwired: 1 in]
      }
      frame 1 {
        n138 = Bundle("AI Y before chamber plot"=w175, "AI Y before chamber plot"=w175) -> (w176:T13)  [unwired: 1 in]
      }
    }
    "AI1" <- w82
  }
  n139 = xnode "Close FPGA VI Reference"("FPGA VI Reference In"=w8, "error in"=w1) -> ("error out"=w7:errorcluster)
  n140 = call <vilib>:"Simple Error Handler.vi"("error in (no error)"=w7) -> ()  [unwired: 4 in, 5 out]
